vi "Scale deaktivieren.vi"(8 "error in (no error)":errorcluster caption="Fehler (Eingang, kein Fehler)", 9 "Autoscale einzeln":bool[](array[boolean]), 10 "Y Anzeige MAX":refnum<vi>[](array[refnum]), 11 "Y Anzeige MIN":refnum<vi>[](array[refnum])) -> (0 "error out":errorcluster caption="Fehler (Ausgang)")   [LabVIEW 2020, in "Grafik.lvlib"]
uses:
  Grafik.lvlib
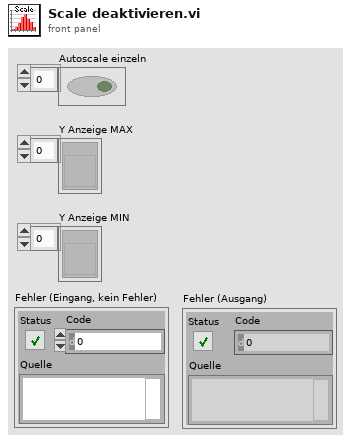
[diagram p1: front panel]
types:
  T1 = enum8{"Enabled", "Disabled", "Disabled and Grayed Out"}
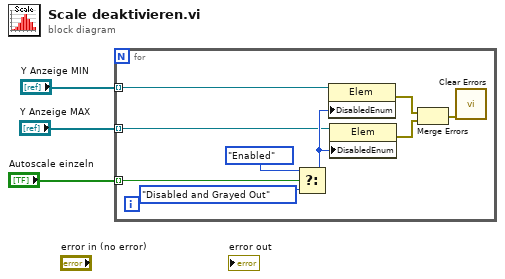
[diagram p0: block diagram]
diagram:
  n1 = for {
    tunnel: "Y Anzeige MIN" -> [w12] mode=indexing
    tunnel: "Y Anzeige MAX" -> [w8] mode=indexing
    tunnel: "Autoscale einzeln" -> [w7] mode=indexing
    n2 = Select(t=T1."Enabled", s=w7, f=T1."Disabled and Grayed Out" ("Deaktiviert")) -> (s? t:f=w9:T1)
    n3 = property class="Elem"(reference=w12, "DisabledEnum"=w9) -> (error out=w6:errorcluster)  [unwired: 1 in, 1 out]
    n4 = property class="Elem"(reference=w8, "DisabledEnum"=w9) -> (error out=w5:errorcluster)  [unwired: 1 in, 1 out]
    n5 = Merge Errors(w6, w5) -> (w4:errorcluster)
    n6 = call <vilib>:"Clear Errors.vi"("error in (no error)"=w4) -> ()  [unwired: 5 in, 2 out]
  }
